vi "Configure Module.vi"(8 "error in (no error)":errorcluster, 10 "IOV ref in":refnum<k21>, 11 "Module Template in":refnum<class "9402.lvclass">) -> (0 "error out":errorcluster, 2 "IOV ref out":refnum<k21>, 3 "Module Template out":refnum<class "9402.lvclass">)   [LabVIEW 2011, in "Modules.lvlib" / "9402.lvclass"]
uses:
  9402.lvclass
  9402.lvclass/9402.ctl
  SD Module/SD Module.lvclass
  Program Files (x86)/National Instruments/LabVIEW 2011/resource/objmgr/cRIO.rc
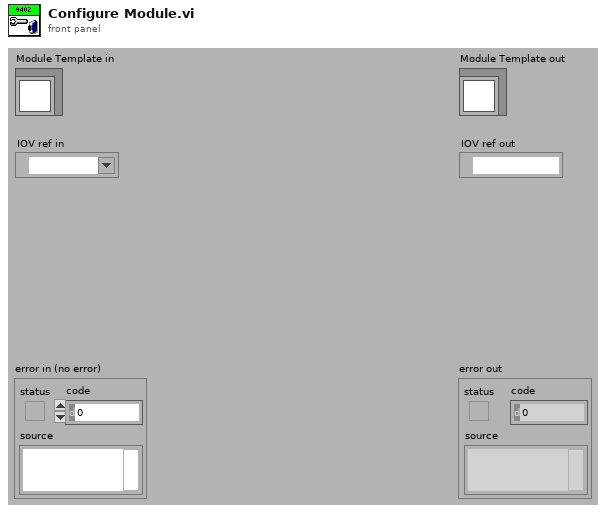
[diagram p1: front panel]
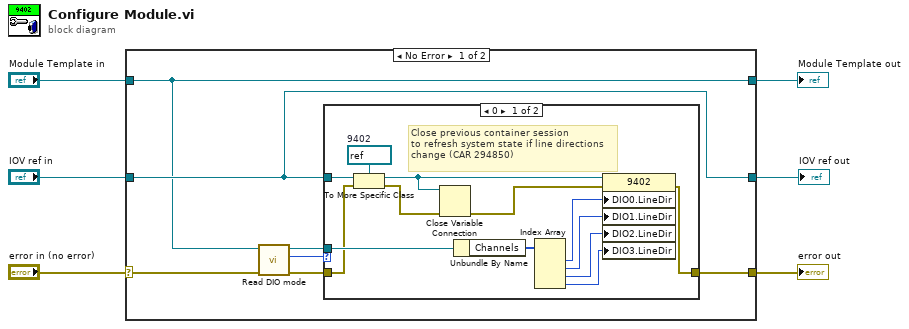
[diagram p0: block diagram]
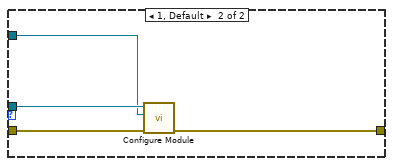
[diagram p2: hidden frame]
diagram:
  n1 = case shown="No Error" "error in (no error)" {
    selector: "error in (no error)" -> [w9 w33]
    tunnel: [w13 w33] -> w5
    tunnel: [w11 w32] -> w3
    tunnel: "Module Template in" -> [w11 w32]
    tunnel: "IOV ref in" -> [w12 w31]
    tunnel: [w12 w31] -> w1
    frame No Error {
      n2 = call "Read DIO mode.vi"("error in (no error)"=w9, "SD Module in"=w11) -> ("error out"=w8:errorcluster, "DIO mode"=w7:u32, "SD Module out"=w10:refnum<class "9402.lvclass">)  [unwired: 7 in]
      n3 = case shown="0" w7 {
        tunnel: [w25 w27] -> w13
        tunnel: w12 -> [w24 w29]
        tunnel: w10 -> [w15 w30]
        tunnel: w8 -> [w14 w28]
        frame 0 {
          w26 = refnum<k21> refnum  # 9402
          # "Close previous container session\nto refresh system state if line directions\nchange (CAR 294850)"
          n4 = To More Specific Class(target class=w26, reference=w24, error in=w14) -> (specific class reference=w18:refnum<k21>, error out=w17:errorcluster)
          n5 = Close Variable Connection(8:w17, 11:w18) -> (0:w16:errorcluster)
          n6 = Unbundle By Name(w15) -> ("Channels"=w23:u32[])
          n7 = Index Array(array=w23) -> (element #1=w22:u32, element #2=w21:u32, element #3=w20:u32, element #4=w19:u32)  [unwired: 4 in]
          n8 = property class="9402"(reference=w18, error in=w16, "DIO0.LineDir"=w22, "DIO1.LineDir"=w21, "DIO2.LineDir"=w20, "DIO3.LineDir"=w19) -> (error out=w25:errorcluster)  [unwired: 1 out]
        }
        frame 1, Default {
          n9 = call-parent "Configure Module.vi"("error in (no error)"=w28, "IOV ref in"=w29, "Module Template in"=w30) -> ("error out"=w27:errorcluster)  [unwired: 6 in, 2 out]
        }
      }
    }
    frame Error {
    }
  }
  "error out" <- w5
  "Module Template out" <- w3
  "IOV ref out" <- w1
